vi "TesteMecanismosControle.vi"   [LabVIEW 2023]
uses:
  <vilib>/Rock Robotics/WPI/RobotDrive/WPI_RobotDriveArcadeDrive_Standard(NoSaturation).vi
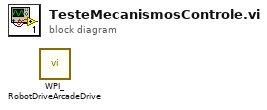
[diagram p0: block diagram]
diagram:
  n1 = call-poly <vilib>:"WPI_RobotDriveArcadeDrive.vi"() -> ()  [unwired: 9 in, 3 out]
